vi "ParseSSHPort.vi"(8 "String in":string, 11 "SSH Login":T1) -> (0 "port":T1, 2 "short name":string, 3 "Full String out":string)   [LabVIEW 2021]
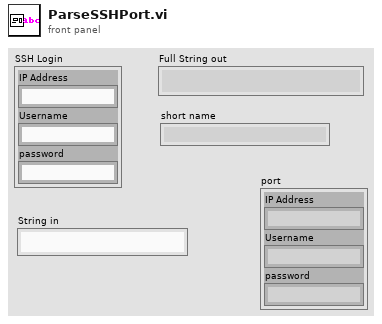
[diagram p1: front panel]
types:
  T1 = cluster{"IP Address":string, "Username":string, "password":string}
  T2 = cluster{"String in":string, "String in":string, "String in":string}
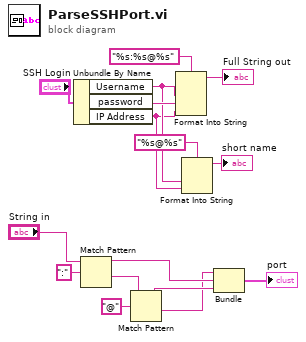
[diagram p0: block diagram]
diagram:
  n1 = Unbundle By Name("SSH Login") -> ("Username"=w3:string, "password"=w15:string, "IP Address"=w2:string)
  n2 = Match Pattern(string="String in", regular expression=":" ("search string/char (-)")) -> (before substring=w7:string, after substring=w8:string)  [unwired: 1 in, 2 out]
  n3 = Match Pattern(string=w8, regular expression="@" ("search string/char (-)")) -> (before substring=w6:string, after substring=w5:string)  [unwired: 1 in, 2 out]
  n4 = Format Into String(format string="%s:%s@%s", w3, w15, w2) -> (resulting string=→"Full String out":string)  [unwired: 2 in, 1 out]
  n5 = Format Into String(format string="%s@%s", w3, w2) -> (resulting string=→"short name":string)  [unwired: 2 in, 1 out]
  n6 = Bundle("String in"=w5, "String in"=w7, "String in"=w6) -> (→"port":T2)  [unwired: 1 in]
